vi "Get LVObject.vi"(8 "error in (no error)":errorcluster, 9 "Object Type":refnum<class>, 10 "Offset":i32, 11 "JSON String containing Flattened Object":string) -> (0 "error out":errorcluster, 1 "Object out":refnum<class>, 2 "Offset past match":i32)   [LabVIEW 2017, in "JSONtext.lvlib"]
doc: "Gets LabVIEW Object that has been flattened and stored as a JSON String."
uses:
  JSONtext.lvlib
  Parsing/Advance past String.vi
  String Subset.vi
  Strip Quotes and Unescape.vi
  Unescape JSON string.vi
  Parsing/Parsing Error.vi
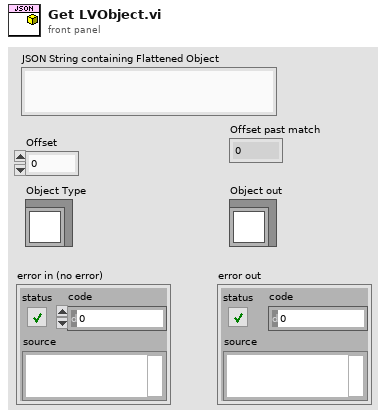
[diagram p1: front panel]
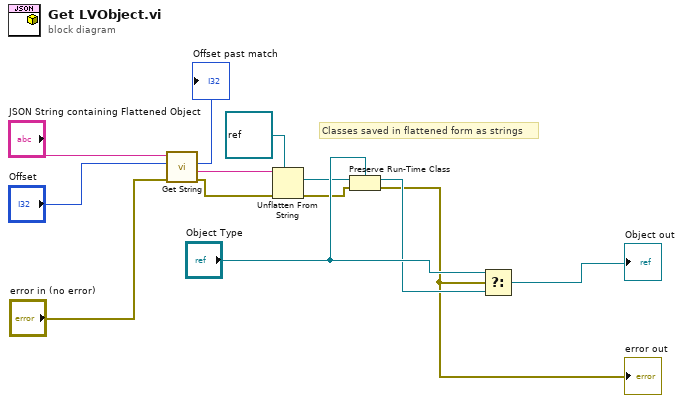
[diagram p0: block diagram]
diagram:
  # "Classes saved in flattened form as strings"
  n1 = call "Get String.vi"("error in (no error)"="error in (no error)", "Offset"="Offset", "JSON"="JSON String containing Flattened Object") -> ("error out"=w12:errorcluster, "String"=w5:string, "Offset past match"=→"Offset past match":i32)  [unwired: 6 in]
  n2 = Unflatten From String(type=refnum<class> refnum ("LabVIEW Object"), binary string=w5, error in (no error)=w12) -> (value=w6:refnum<class>, error out=w7:errorcluster)  [unwired: 2 in, 1 out]
  n3 = Preserve Run-Time Class(object in=w6, error in=w7, 2:"Object Type") -> (object out=w9:refnum<class>, error out=w8:errorcluster)
  "error out" <- w8
  n4 = Select(t="Object Type", s=w8, f=w9) -> (s? t:f=→"Object out":refnum<class>)
